vi "Main_4_Dynamic[FPGA].vi"() -> ()   [LabVIEW 2017]
uses:
  <vilib>/LabVIEW Targets/FPGA/cRIO/shared/nicrio_ModuleControls/nicrio_cRIO-9232_ConfigModeRing.ctl
  <vilib>/rvi/Emulation/niFpgaGetClockAttributes.vi
  <vilib>/rvi/Emulation/niFpgaSctlEmulationGetInTimedLoop.vi
  <vilib>/rvi/Emulation/niFpgaEmulationReportErrorSimple.vi
  <vilib>/rvi/Emulation/niFpgaProcessEmulError.vi
  <vilib>/rvi/eio/common/nirviEmuTemplateMethod_errors.vi
  <vilib>/rvi/interface/RandomDataEmulation/niFpgaRandomDataHandleErrors.vi
  <vilib>/rvi/Emulation/niFpgaCriticalErrorInLSC.vi
  <vilib>/eio/EIONode/EIONode.xnode
  <vilib>/rvi/DataTransferAndStorage/Container/XNode/niFpgaContainer.xnode
  <vilib>/rvi/interface/RandomDataEmulation/nirviRandomDataFpgaReadWriteTemplate.vi
  <vilib>/addons/InsightCM/Devices/Shared/Cms/Fpga/Acquisition/source/subVIs/VibAPI_4/BOP_VibAPI_4.lvlib
panel:
  out "Chassis Temperature":sgl
  in  "Custom Scale Intercept":sgl[](array[numeric])=[0.0, 0.0, 0.0, 0.0, 0.0, 0.0, 0.0, 0.0, 0.0, 0.0, 0.0, 0.0, 0.0, 0.0, 0.0, 0.0, 0.0, 0.0, 0.0, 0.0, 0.0, 0.0, 0.0, 0.0, 0.0, 0.0, 0.0, 0.0, 0.0, 0.0, 0.0, 0.0]
  out "FPGA Error":errorcluster
  out "Finished":bool
  in  "Stop":bool
  out "Module Underflow":bool
  out "DMA FIFO Full":bool
  out "Chan Count":bool
  out "Acq Loop Ticks":u32
  out "Short Circuit Chan Array":bool[](array[boolean])
  out "Open Loop Chan Array":bool[](array[boolean])
  out "First Read":bool
  in  "Total Avail Channels":i32=4
  in  "Data Rate [S/s]":u32=1280
  in  "Custom Scale Slope":sgl[](array[numeric])=[0.0, 0.0, 0.0, 0.0, 0.0, 0.0, 0.0, 0.0, 0.0, 0.0, 0.0, 0.0, 0.0, 0.0, 0.0, 0.0, 0.0, 0.0, 0.0, 0.0, 0.0, 0.0, 0.0, 0.0, 0.0, 0.0, 0.0, 0.0, 0.0, 0.0, 0.0, 0.0]
  in  "Acquisition Type":enum16{"Finite Samples", "Continuous Samples"}(ring)
  in  "Samps per Chan [Finite]":i32=5120
  in  "Input Config Array":T1[](array[typedef])=[0, 0, 0, 0, 0, 0, 0, 0, 0, 0, 0, 0, 0, 0, 0, 0, 0, 0, 0, 0, 0, 1, 1, 1, 0, 0, 0, 0, 0, 0, 0, 0] items=["AC Coupled", "DC Coupled", "IEPE AC Coupled"]
  in  "Number of Modules":i16=1
  in  "Enable Chan Array":bool[](array[boolean])=[FALSE, FALSE, FALSE, FALSE, FALSE, FALSE, FALSE, FALSE, FALSE, FALSE, FALSE, FALSE, FALSE, FALSE, FALSE, FALSE, FALSE, FALSE, FALSE, FALSE, FALSE, FALSE, FALSE, FALSE, FALSE, FALSE, FALSE, FALSE, FALSE, FALSE, FALSE, FALSE]
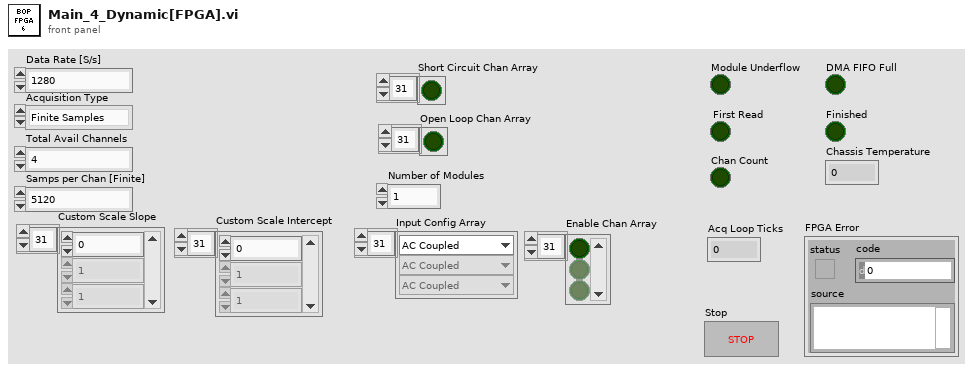
[diagram p1: front panel]
types:
  T1 = typedef "nicrio_cRIO-9232_ConfigModeRing.ctl" = u8
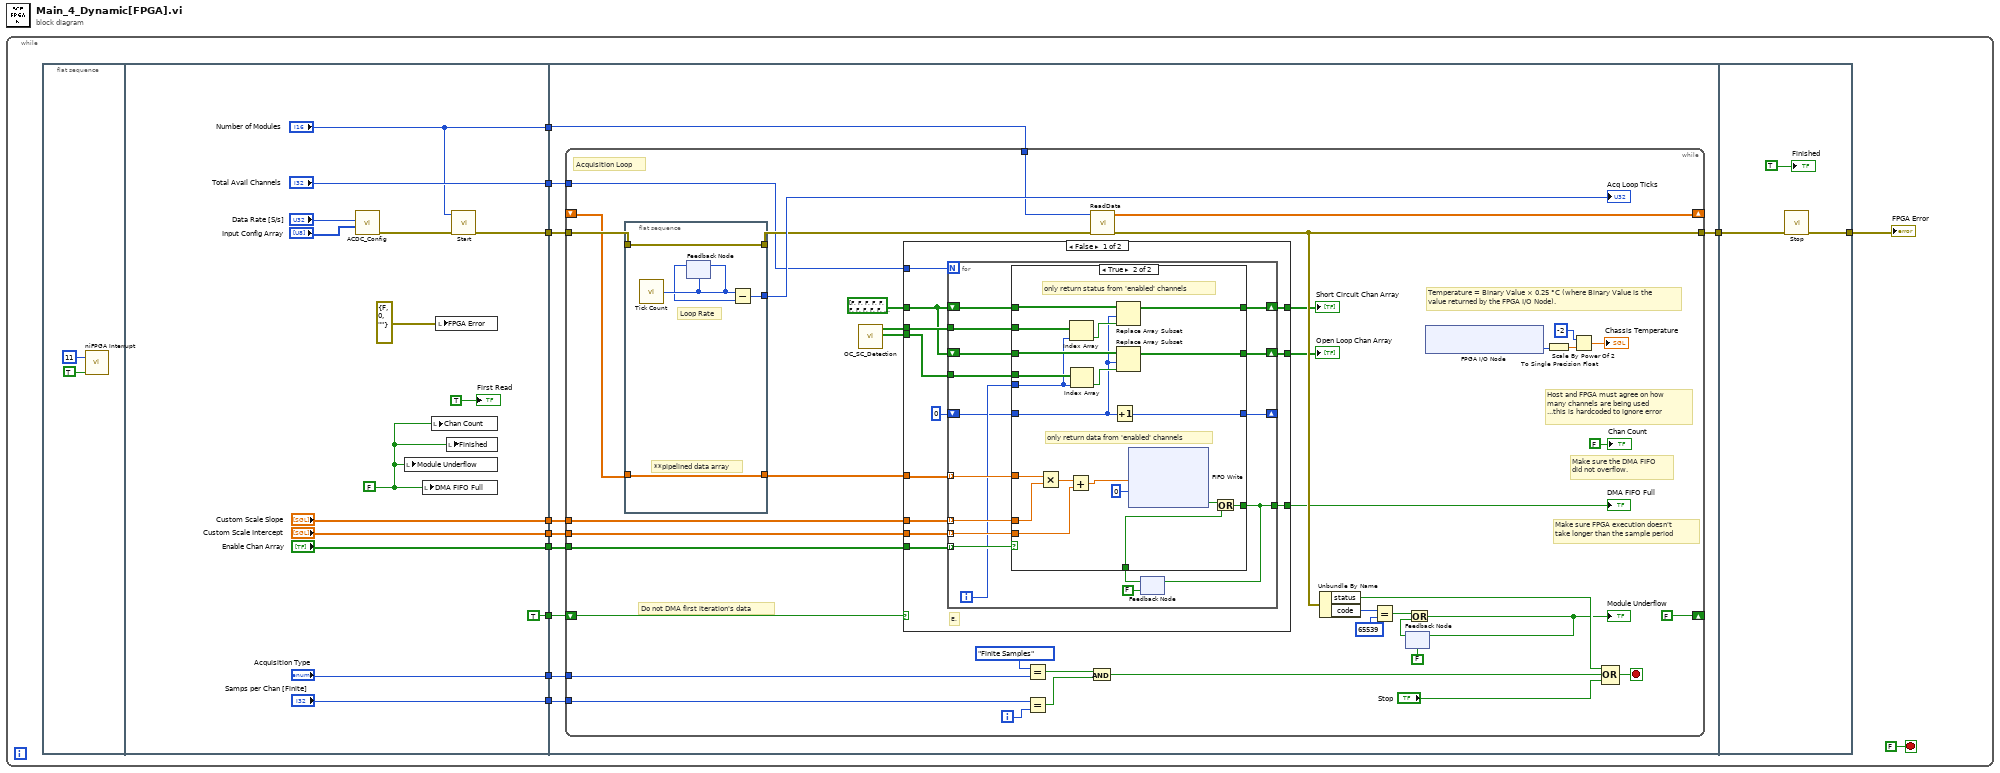
[diagram p0: block diagram]
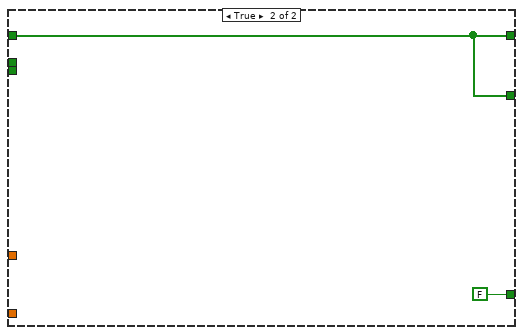
[diagram p3: hidden frame]
diagram:
  n1 = while {
    stop <- FALSE stop-if-true
    n2 = flat-sequence {
      tunnel: [w22] -> w11
      tunnel: ["Custom Scale Slope"] -> w10
      tunnel: ["Acquisition Type"] -> w9
      tunnel: ["Samps per Chan [Finite]"] -> w8
      tunnel: ["Total Avail Channels"] -> w7
      tunnel: [TRUE ("t")] -> w6
      tunnel: ["Number of Modules"] -> w4
      tunnel: ["Enable Chan Array"] -> w3
      tunnel: ["Custom Scale Intercept"] -> w1
      tunnel: w11 -> [w38]
      tunnel: w10 -> [w37]
      tunnel: w9 -> [w35]
      tunnel: w8 -> [w34]
      tunnel: w7 -> [w39]
      tunnel: w6 -> [w36]
      tunnel: [w33] -> w5
      tunnel: w4 -> [w32]
      tunnel: w3 -> [w31]
      tunnel: w1 -> [w30]
      tunnel: w5 -> [w141]
      tunnel: [w140] -> w2
      frame #0 {
        n3 = call <vilib>:"niFPGA Interrupt.vi"("Wait Until Cleared (F)"=TRUE ("Wait Until Cleared"), "IRQ Number (0)"=u8 11 ("IRQ Number")) -> ()  [unwired: 1 in]
      }
      frame #1 {
        w23 = FALSE ("Module Underflow")
        n4 = call <vilib>:"ACDC_Config.vi"("Input Config Array"="Input Config Array", "Data Rate [S/s]"="Data Rate [S/s]") -> ("error out"=w20:errorcluster)  [unwired: 9 in]
        n5 = local write "Module Underflow"(w23) -> ()
        n6 = local write "DMA FIFO Full"(w23) -> ()
        n7 = local write "Chan Count"(w23) -> ()
        n8 = local write "FPGA Error"(errorcluster {"status"=FALSE, "code"=0, "source"=""} ("FPGA Error")) -> ()
        n9 = local write "Finished"(w23) -> ()
        n10 = call <vilib>:"Start.vi"("error in (no error)"=w20, "Module Config Selector"="Number of Modules") -> ("error out"=w22:errorcluster)  [unwired: 9 in]
        "First Read" <- TRUE ("First Read")
      }
      frame #2 {
        n11 = while {
          tunnel: w38 -> [w73]
          tunnel: [w74] -> w33
          tunnel: w35 -> [w76]
          tunnel: w34 -> [w75]
          shift-right: [w68] -> _
          shift-left: _ -> [w71]
          tunnel: w39 -> [w52]
          tunnel: w37 -> [w51]
          shift-right: [FALSE ("t")] -> _
          shift-left: w36 -> [w55]
          tunnel: w32 -> [w58]
          tunnel: w31 -> [w50]
          tunnel: w30 -> [w49]
          i -> [w69]
          stop <- w79 stop-if-true
          # "Temperature = Binary Value × 0.25 °C (where Binary Value is the value returned by the FPGA I/O Node)."
          # "Do not DMA first iteration's data"
          # "Acquisition Loop"
          # "Host and FPGA must agree on how \nmany channels are being used\n...this is hardcoded to ignore error"
          # "Make sure the DMA FIFO\ndid not overflow."
          # "Make sure FPGA execution doesn't\ntake longer than the sample period"
          n12 = flat-sequence {
            tunnel: [w139] -> w56
            tunnel: w73 -> [w139]
            tunnel: [w136] -> w72
            tunnel: w71 -> [w135]
            tunnel: [w135] -> w53
            frame #0 {
              # "**pipelined data array"
              # "Loop Rate"
              n13 = call "Tick Count"() -> ("Tick Count(Ticks)"=w138:u32)
              n14 = feedback-in #1(w138) -> ()
              n15 = feedback #1(w138) -> (w137:u32)
              n16 = Subtract(x=w138, y=w137) -> (x-y=w136:u32)
            }
          }
          n17 = call <vilib>:"OC_SC_Detection.vi"() -> ("Open Loop Channels Array"=w47:bool[], "Short Circuit Channels Array"=w48:bool[])  [unwired: 10 in]
          n18 = case shown="False" w55 {
            tunnel: [w92 FALSE] -> w54
            tunnel: w51 -> [w91 _]
            tunnel: w53 -> [w90 _]
            tunnel: w52 -> [w89 _]
            tunnel: w50 -> [w88 _]
            tunnel: w49 -> [w87 _]
            tunnel: w48 -> [w86 _]
            tunnel: w47 -> [w85 _]
            tunnel: bool[] [FALSE, FALSE, FALSE, FALSE, FALSE, FALSE, FALSE, FALSE, FALSE, FALSE, FALSE, FALSE, FALSE, FALSE, FALSE, FALSE, FALSE, FALSE, FALSE, FALSE, FALSE, FALSE, FALSE, FALSE, FALSE, FALSE, FALSE, FALSE, FALSE, FALSE, FALSE, FALSE] ("Open Loop Chan Array") -> [w84 w133]
            tunnel: [w83 w133] -> w45
            tunnel: [w82 w133] -> w44
            frame False {
              # "E."
              n19 = for {
                N: w89 -> [_]
                tunnel: [w107] -> w92
                tunnel: w90 -> [w106] mode=indexing
                tunnel: w91 -> [w105] mode=indexing
                tunnel: w88 -> [w103] mode=indexing
                tunnel: w87 -> [w102] mode=indexing
                tunnel: w86 -> [w96]
                tunnel: w85 -> [w97]
                shift-right: [w99] -> w83
                shift-left: w84 -> [w100]
                shift-right: [w98] -> w82
                shift-left: w84 -> [w101]
                shift-right: [w93] -> _
                shift-left: 0 -> [w94]
                i -> [w95]
                n20 = feedback #2(FALSE) -> (w108:bool)
                n21 = case shown="True" w103 {
                  tunnel: w108 -> [w112 w132]
                  tunnel: [w112 w131] -> w107
                  tunnel: w106 -> [_ w130]
                  tunnel: w105 -> [_ w129]
                  tunnel: w102 -> [_ w124]
                  tunnel: w101 -> [w110 w121]
                  tunnel: w100 -> [w111 w120]
                  tunnel: [w111 w119] -> w99
                  tunnel: [w110 w118] -> w98
                  tunnel: w97 -> [_ w117]
                  tunnel: w96 -> [_ w116]
                  tunnel: w95 -> [_ w115]
                  tunnel: w94 -> [w109 w114]
                  tunnel: [w109 w113] -> w93
                  frame False {
                  }
                  frame True {
                    # "only return status from 'enabled' channels"
                    # "only return data from 'enabled' channels"
                    n22 = Multiply(x=w130, y=w129) -> (x*y=w126:sgl)
                    n23 = Add(x=w126, y=w124) -> (x+y=w125:sgl)
                    n24 = Index Array(array=w116, index=w115) -> (element=w123:bool)
                    n25 = Index Array(array=w117, index=w115) -> (element=w122:bool)
                    n26 = Increment(x=w114) -> (x+1=w113:i32)
                    n27 = Replace Array Subset(array=w120, new element=w123, index=w114) -> (w119:bool[])
                    n28 = Replace Array Subset(array=w121, new element=w122, index=w114) -> (w118:bool[])
                    n29 = xnode ("FIFO Write")("Element"=w125, "Timeout"=0) -> ("Timed Out?"=w127:bool)  [unwired: 1 in, 1 out]
                    n30 = Or(x=w127, y=w132) -> (x .or. y?=w131:bool)
                  }
                }
                n31 = feedback-in #2(w107) -> ()
              }
            }
            frame True {
            }
          }
          "DMA FIFO Full" <- w54
          "Short Circuit Chan Array" <- w45
          "Open Loop Chan Array" <- w44
          n32 = Equal?(x=enum16{"Finite Samples", "Continuous Samples"}."Finite Samples" ("y"), y=w76) -> (x = y?=w62:bool)
          n33 = Equal?(x=w75, y=w69) -> (x = y?=w61:bool)
          n34 = And(x=w62, y=w61) -> (x .and. y?=w60:bool)
          n35 = call <vilib>:"ReadData.vi"("error in"=w56, "Module Config Selector"=w58) -> ("error out"=w74:errorcluster, "Data Array"=w68:sgl[])  [unwired: 8 in]
          n36 = Unbundle By Name(w74) -> ("status"=w67:bool, "code"=w77:i32)
          n37 = Equal?(x=w77, y=65539) -> (x = y?=w64:bool)
          n38 = feedback #3(FALSE) -> (w66:bool)
          n39 = Or(x=w64, y=w66) -> (x .or. y?=w63:bool)
          "Module Underflow" <- w63
          n40 = feedback-in #3(w63) -> ()
          n41 = xnode "FPGA I/O Node"() -> ("Chassis Temperature"=w41:i16)  [unwired: 1 in, 1 out]
          n42 = To Single Precision Float(number=w41) -> (single precision float=w43:sgl)
          n43 = Scale By Power Of 2(n=i16 -2, x=w43) -> (x*2^n=→"Chassis Temperature":sgl)
          n44 = Compound Arithmetic op=OR(w67, w60, "Stop") -> (w79:bool)
          "Chan Count" <- FALSE ("Chan Count")
          "Acq Loop Ticks" <- w72
        }
      }
      frame #3 {
        n45 = call <vilib>:"Stop.vi"("error in (no error)"=w141) -> ("error out"=w140:errorcluster)  [unwired: 10 in]
        "Finished" <- TRUE ("Finished")
      }
    }
    "FPGA Error" <- w2
  }
